vi "ModifiedBasicFGen.vi"(0 "frequency":dbl=10.0 format="%0.2p", 1 "signal type":T1(ring), 2 "reset time":bool, 5 "amplitude":dbl=1.0 format="%0.2p", 7 "phase":dbl format="%.2p", 9 "tf in":timestamp, 11 "error in (no error)":errorcluster, 12 "offset":dbl format="%0.2p", 13 "square wave duty cycle (%)":dbl=50.0 format="%0.2f", 14 "sampling info":cluster{"Fs":dbl, "#s":dbl}={"Fs"=1000.0, "#s"=1000.0} {"Fs" format="%.2p"}) -> (4 "signal out":waveform(dbl), 8 "phase out":dbl format="%.2p", 10 "tf out":timestamp, 15 "error out":errorcluster)   [LabVIEW 2023]
uses:
  <vilib>/measure/maUtilsandCtls.llb/ma_Updatet0 timestamp.vi
  <vilib>/measure/NI_MABase.lvlib
  <vilib>/Analysis/NI_AALBase.lvlib
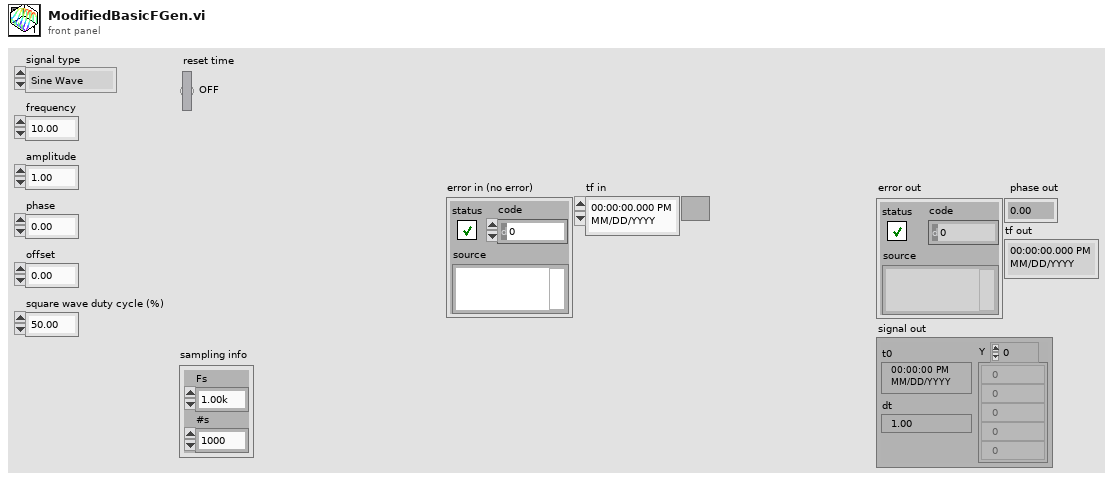
[diagram p1: front panel]
types:
  T1 = enum16{"Sine Wave", "Triangle Wave", "Square Wave", "Sawtooth Wave"}
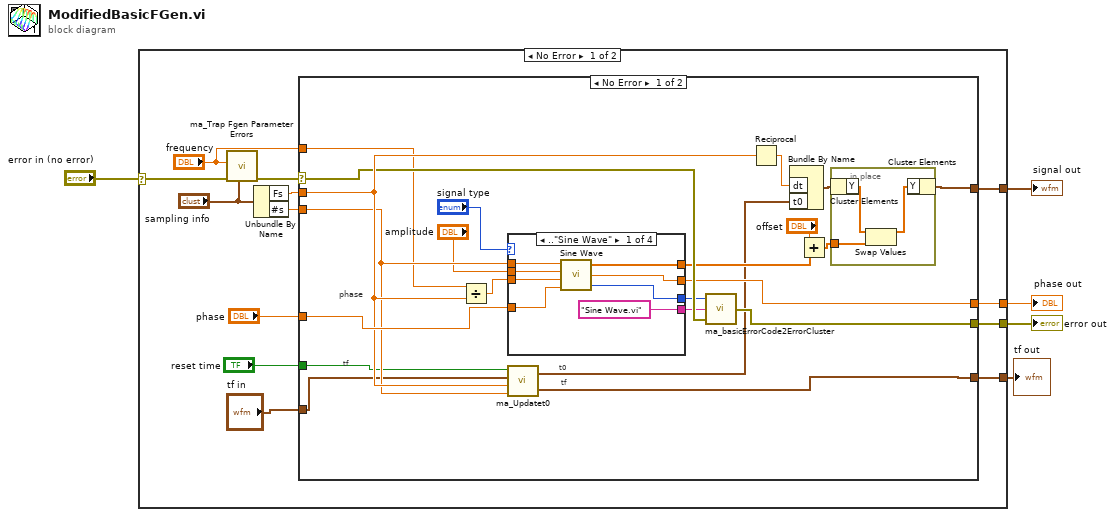
[diagram p0: block diagram]
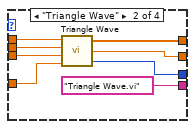
[diagram p2: hidden frame]
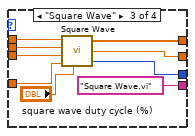
[diagram p3: hidden frame]
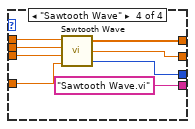
[diagram p4: hidden frame]
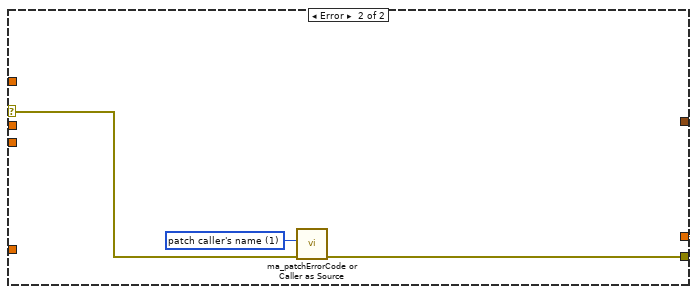
[diagram p5: hidden frame]
diagram:
  n1 = case shown="No Error" "error in (no error)" {
    selector: "error in (no error)" -> [w12 w81]
    tunnel: [w18 w81] -> w5
    tunnel: [w10 _] -> w3
    tunnel: [w9 _] -> w2
    tunnel: [w7 _] -> w1
    frame No Error {
      n2 = call <vilib>:"ma_Trap Fgen Parameter Errors.vi"("Sampling info"="sampling info", "error in (no error)"=w12, "frequency"="frequency") -> ("error out"=w17:errorcluster)  [unwired: 8 in]
      n3 = Unbundle By Name("sampling info") -> ("Fs"=w14:dbl, "#s"=w13:dbl)
      n4 = case shown="No Error" w17 {
        selector: w17 -> [w36 w79]
        tunnel: [w30 w80] -> w9
        tunnel: [w40 w78] -> w18
        tunnel: "phase" -> [w39 _]
        tunnel: w14 -> [w38 _]
        tunnel: w13 -> [w37 _]
        tunnel: [w34 _] -> w10
        tunnel: "frequency" -> [w35 _]
        tunnel: "reset time" -> [w33 _]
        tunnel: [w32 _] -> w7
        tunnel: "tf in" -> [w31 _]
        frame No Error {
          # "tf"
          # "t0"
          # "phase"
          # "tf"
          n5 = Divide(x=w35, y=w38) -> (x/y=w28:dbl)
          n6 = case shown="..\"Sine Wave\"" "signal type" {
            tunnel: w28 -> [w51 w59 w68 w76]
            tunnel: "amplitude" -> [w50 w58 w67 w75]
            tunnel: w37 -> [w49 w57 w66 w74]
            tunnel: w39 -> [w48 w56 w65 w73]
            tunnel: [w47 w55 w64 w72] -> w30
            tunnel: [w46 w54 w63 w71] -> w27
            tunnel: ["Sine Wave.vi" ("subVI Name") "Triangle Wave.vi" ("subVI Name") "Square Wave.vi" ("subVI Name") "Sawtooth Wave.vi" ("subVI Name")] -> w24
            tunnel: [w45 w53 w61 w69] -> w23
            frame .."Sine Wave" {
              n7 = call <vilib>:"Sine Wave.vi"("samples"=w49, "amplitude"=w50, "frequency"=w51, "phase in"=w48) -> ("sine wave"=w46:dbl[], "phase out"=w47:dbl, "error"=w45:i32)  [unwired: 1 in]
            }
            frame "Triangle Wave" {
              n8 = call <vilib>:"Triangle Wave.vi"("samples"=w57, "amplitude"=w58, "frequency"=w59, "phase in"=w56) -> ("triangle wave"=w54:dbl[], "phase out"=w55:dbl, "error"=w53:i32)  [unwired: 1 in]
            }
            frame "Square Wave" {
              n9 = call <vilib>:"Square Wave.vi"("samples"=w66, "amplitude"=w67, "frequency"=w68, "duty cycle (%)"="square wave duty cycle (%)", "phase in"=w65) -> ("square wave"=w63:dbl[], "phase out"=w64:dbl, "error"=w61:i32)  [unwired: 1 in]
            }
            frame "Sawtooth Wave" {
              n10 = call <vilib>:"Sawtooth Wave.vi"("samples"=w74, "amplitude"=w75, "frequency"=w76, "phase in"=w73) -> ("sawtooth wave"=w71:dbl[], "phase out"=w72:dbl, "error"=w69:i32)  [unwired: 1 in]
            }
          }
          n11 = call-poly <vilib>:"ma_Updatet0.vi"("samples"=w37, "sampling rate (S/s)"=w38, "tf previous"=w31, "Reset Generation"=w33) -> ("tf new"=w32:timestamp, "t0"=w22:timestamp)
          n12 = call <vilib>:"ma_basicErrorCode2ErrorCluster.vi"("error in (no error)"=w36, "subVI name"=w24, "Error Code"=w23) -> ("error out"=w40:errorcluster)
          n13 = Reciprocal(x=w38) -> (1/x=w29:dbl)
          n14 = Bundle By Name("dt"=w29, "t0"=w22) -> (w19:waveform(dbl))  [unwired: 1 in]
          n15 = Add(x="offset", y=w27) -> (x+y=w20:dbl[])
          n16 = in-place {
            in-place-border: w20 -> [w41]
            n17 = in-place-cluster #1(w19) -> ("Y"=w43:dbl[])
            n18 = Swap Values(12:w43, 14:w41) -> (1:w42:dbl[])  [unwired: 1 in, 1 out]
            n19 = in-place-cluster #1("Y"=w42) -> (w34:waveform(dbl))
          }
        }
        frame Error {
          w77 = u16 1 items=["patch error code", "patch caller's name"] ("operation")
          w80 = 0.0  # phase out
          n20 = call <vilib>:"ma_patchErrorCode or Caller as Source.vi"("error in (no error)"=w79, "operation"=w77) -> ("error out"=w78:errorcluster)  [unwired: 9 in]
        }
      }
    }
    frame Error {
    }
  }
  "error out" <- w5
  "signal out" <- w3
  "phase out" <- w2
  "tf out" <- w1
